vi "Create Oneof Message Converter Skeletons.vi"(8 "error in (no error)":errorcluster, 10 "Message parameters":T1[](array[typedef]), 11 "Library in":refnum<vi>) -> (0 "error out":errorcluster, 3 "Library out":refnum<vi>)   [LabVIEW 2025, in "gRPC Template Creation Utility.lvlib"]
uses:
  gRPC Template Creation Utility.lvlib
  TypeDefs/Message Metadata (Scripting).ctl
  TypeDefs/Message Element Metadata (Scripting).ctl
  TypeDefs/Message Element Type.ctl
  OneOf Constants/OneOfConstantsEnum.ctl
  <vilib>/Utility/traverseref.llb/TRef TravTarget.ctl
  <vilib>/Utility/traverseref.llb/VI Scripting - Traverse.lvlib
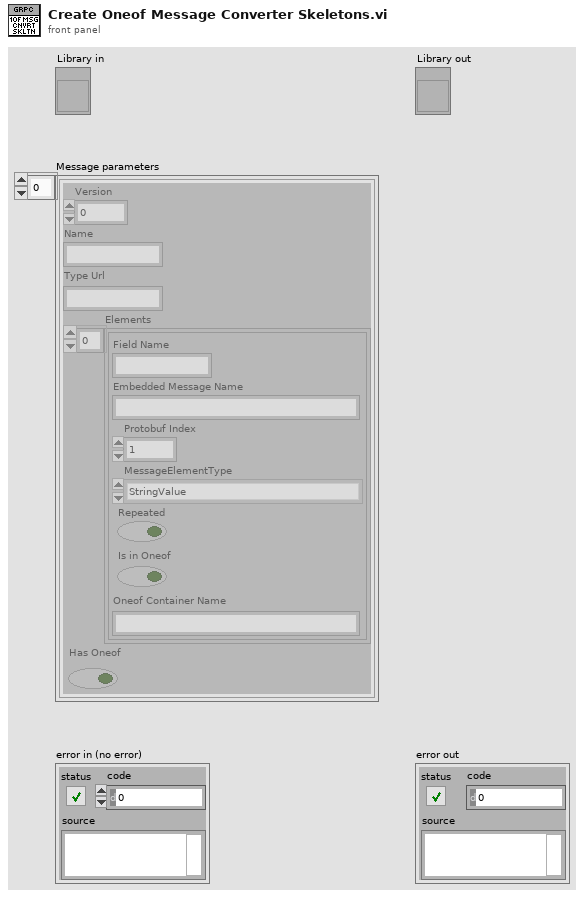
[diagram p1: front panel]
types:
  T1 = typedef "gRPC Template Creation Utility.lvlib/Message Metadata (Scripting).ctl" = cluster{"Version":i32, "Name":string, "Type Url":string, "Elements":T2[], "Has Oneof":bool}
  T2 = typedef "gRPC Template Creation Utility.lvlib/Message Element Metadata (Scripting).ctl" = cluster{"Field Name":string, "Embedded Message Name":string, "Protobuf Index":i32, "MessageElementType":T3, "Repeated":bool, "Is in Oneof":bool, "Oneof Container Name":string}
  T3 = typedef "gRPC Template Creation Utility.lvlib/Message Element Type.ctl" = enum32{"Int32Value", "FloatValue", "DoubleValue", "BoolValue", "StringValue", "MessageValue", "Int64Value", "UInt32Value", "UInt64Value", "EnumValue", "Bytes", "Fixed64", "Fixed32", "SFixed64", "SFixed32", "SInt64", "SInt32"}
  T4 = typedef "gRPC Template Creation Utility.lvlib/OneOfConstantsEnum.ctl" = enum16{"FlatToRichVIPrefix", "RichToFlatVIPrefix", "FlatTypeDefSuffix"}
  T5 = typedef "TRef TravTarget.ctl" = enum16{"FP", "BD", "Other"}
  T6 = enum32{"invalid scope", "public", "private", "protected", "community"}
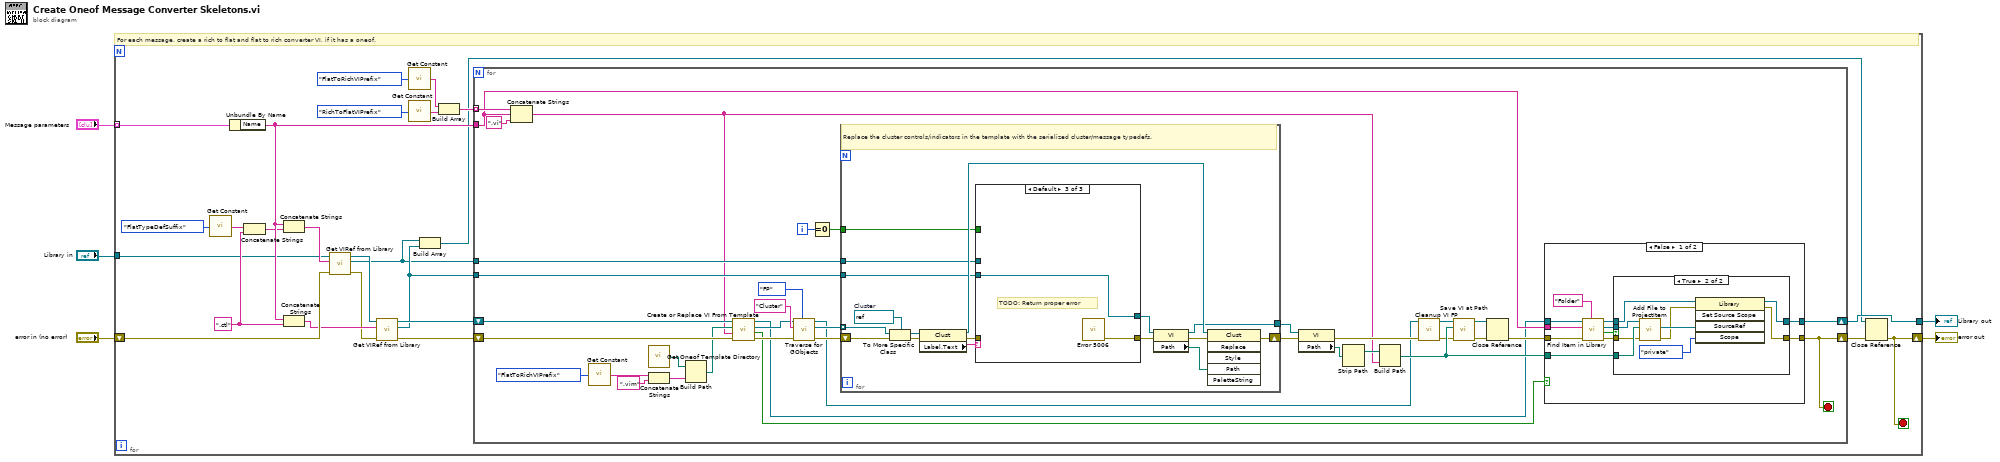
[diagram p0: block diagram]
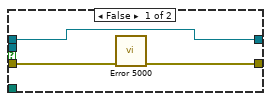
[diagram p2: hidden frame]
diagram:
  n1 = for {
    tunnel: "Message parameters" -> [w30] mode=indexing
    shift-right: [w7] -> w3
    shift-left: "error in (no error)" -> [w29]
    tunnel: "Library in" -> [w14]
    tunnel: [w27] -> w5
    stop <- w7 stop-if-true
    w15 = ".ctl" ("string")
    # "For each message, create a rich to flat and flat to rich converter VI, if it has a oneof."
    n2 = call "Get Constant.vi"("Selection"=OneOfConstantsEnum."FlatTypeDefSuffix") -> ("String"=w21:string)
    n3 = Unbundle By Name(w30) -> ("Name"=w24:string)
    n4 = Concatenate Strings(w21, w15) -> (w23:string)
    n5 = Concatenate Strings(w24, w23) -> (w26:string)
    n6 = Concatenate Strings(w24, w15) -> (w25:string)
    n7 = call "Get VIRef from Library.vi"("error in (no error)"=w29, "item name"=w26, "library in"=w14) -> ("error out"=w12:errorcluster, "vi"=w9:refnum<vi>, "library out"=w13:refnum<vi>)  [unwired: 5 in, 1 out]
    n8 = call "Get VIRef from Library.vi"("error in (no error)"=w12, "item name"=w25, "library in"=w13) -> ("error out"=w11:errorcluster, "vi"=w10:refnum<vi>, "library out"=w28:refnum<vi>)  [unwired: 5 in, 1 out]
    n9 = call "Get Constant.vi"("Selection"=OneOfConstantsEnum."FlatToRichVIPrefix") -> ("String"=w18:string)
    n10 = call "Get Constant.vi"("Selection"=OneOfConstantsEnum."RichToFlatVIPrefix") -> ("String"=w17:string)
    n11 = Build Array(w9, w10) -> (w6:refnum<vi>[])
    n12 = Build Array(w18, w17) -> (w16:string[])
    n13 = for {
      tunnel: w9 -> [w68]
      tunnel: w24 -> [w52]
      tunnel: w10 -> [w63]
      shift-right: [w40] -> w27
      shift-left: w28 -> [w35]
      shift-right: [w32] -> w8
      shift-left: w11 -> [w39]
      tunnel: w16 -> [w57] mode=indexing
      i -> [w56]
      stop <- w32 stop-if-true
      n14 = Concatenate Strings(w57, w52, ".vi" ("string")) -> (w33:string)
      n15 = call "Get Constant.vi"("Selection"=OneOfConstantsEnum."FlatToRichVIPrefix") -> ("String"=w50:string)
      n16 = call "Get Oneof Template Directory.vi"() -> ("appended path"=w53:path)
      n17 = Concatenate Strings(w50, ".vim" ("string")) -> (w48:string)
      n18 = Build Path(base path=w53, name or relative path=w48) -> (appended path=w34:path)
      n19 = call "Create or Replace VI From Template.vi"("error in (no error)"=w39, "vi name"=w33, "template vi path"=w34, "library in"=w35) -> ("error out"=w38:errorcluster, "existing vi"=w31:bool, "vi"=w37:refnum<vi>, "Library out"=w36:refnum<vi>)  [unwired: 4 in]
      n20 = call <vilib>:"Traverse for GObjects.vi"("Traverse Target"=TRef_TravTarget."FP", "error in (no error)"=w38, "Class Name"="Cluster", "VI Refnum"=w37) -> ("error out"=w58:errorcluster, "References"=w60:refnum<vi>[], "dup VI Refnum"=w45:refnum<vi>)  [unwired: 4 in, 1 out]
      n21 = Equal To 0?(x=w56) -> (x = 0?=w55:bool)
      n22 = for {
        tunnel: w60 -> [w101] mode=indexing
        tunnel: w68 -> [w105]
        tunnel: w63 -> [w104]
        shift-right: [w100] -> w59
        shift-left: w58 -> [w102]
        tunnel: [w99] -> w67
        tunnel: w55 -> [w94]
        w109 = refnum<vi> refnum  # Cluster
        # "Replace the cluster controls/indicators in the template with the serialized cluster/message typedefs."
        n23 = To More Specific Class(target class=w109, reference=w101, error in=w102) -> (specific class reference=w108:refnum<vi>, error out=w110:errorcluster)
        n24 = property class="Clust"(reference=w108, error in=w110) -> (reference out=w106:refnum<vi>, error out=w103:errorcluster, "Label.Text"=w107:string)
        n25 = case shown="Default" w107 {
          tunnel: w105 -> [w113 w121 _]
          tunnel: w104 -> [w112 w120 w125]
          tunnel: w103 -> [w115 w118 _]
          tunnel: [w111 w119 w125] -> w95
          tunnel: [w115 w118 w126] -> w96
          tunnel: w94 -> [w114 w122 _]
          frame "OutputCluster", "OutputClusterType" {
            n26 = case shown="True" w114 {
              tunnel: w113 -> [w116 _]
              tunnel: w112 -> [_ w117]
              tunnel: [w116 w117] -> w111
              frame False {
                # "Convert Class to Cluster. Wire flat cluster as output"
              }
              frame True {
                # "Convert Cluster to Class.\nWire rich cluster as output"
              }
            }
          }
          frame "InputCluster" {
            n27 = case shown="True" w122 {
              tunnel: w121 -> [_ w124]
              tunnel: w120 -> [w123 _]
              tunnel: [w123 w124] -> w119
              frame False {
                # "Convert Class to Cluster. Wire rich cluster as input."
              }
              frame True {
                # "Convert Cluster to Class. Wire flat cluster as input"
              }
            }
          }
          frame Default {
            # "TODO: Return proper error"
            n28 = call "Error 5006.vi"() -> ("error out"=w126:errorcluster)  [unwired: 11 in]
          }
        }
        n29 = property class="VI"(reference=w95, error in=w96) -> (reference out=w99:refnum<vi>, error out=w98:errorcluster, "Path"=w97:path)
        n30 = invoke class="Clust" method="Replace"(reference=w106, error in=w98, "Path"=w97) -> (error out=w100:errorcluster)  [unwired: 3 in, 5 out]
      }
      n31 = property class="VI"(reference=w67, error in=w59) -> (error out=w47:errorcluster, "Path"=w66:path)  [unwired: 1 out]
      n32 = Strip Path(path=w66) -> (stripped path=w65:path)  [unwired: 1 out]
      n33 = Build Path(base path=w65, name or relative path=w33) -> (appended path=w54:path)
      n34 = call "Cleanup VI FP.vi"("error in"=w47, "vi in"=w45) -> ("error out"=w46:errorcluster, "vi out"=w44:refnum<vi>)  [unwired: 8 in]
      n35 = call "Save VI at Path.vi"("error in (no error)"=w46, "Path"=w54, "VI in"=w44) -> ("error out"=w43:errorcluster, "VI out"=w42:refnum<vi>)  [unwired: 6 in, 1 out]
      n36 = Close Reference(reference=w42, error in (no error)=w43) -> (error out=w41:errorcluster)
      n37 = case shown="False" w31 {
        tunnel: w54 -> [w77 _]
        tunnel: w52 -> [w74 _]
        tunnel: w41 -> [w73 w93]
        tunnel: [w71 w92] -> w40
        tunnel: w36 -> [w70 w92]
        tunnel: [w69 w93] -> w32
        frame False {
          n38 = call "Find Item in Library.vi"("Item Type"="Folder", "error in (no error)"=w73, "Item Name"=w74, "Library item in"=w70) -> ("error out"=w76:errorcluster, "Found?"=w75:bool, "Project Item (Library Item)"=w78:refnum<vi>, "Library item out"=w72:refnum<vi>)  [unwired: 4 in]
          n39 = case shown="True" w75 {
            tunnel: w78 -> [_ w91]
            tunnel: w77 -> [_ w90]
            tunnel: w76 -> [w81 w89]
            tunnel: [w80 w84] -> w69
            tunnel: w72 -> [w82 w88]
            tunnel: [w82 w86] -> w71
            frame False {
              n40 = call "Error 5000.vi"("error in (no error)"=w81) -> ("error out"=w80:errorcluster)  [unwired: 10 in]
            }
            frame True {
              n41 = call "Add File to ProjectItem.vi"("error in (no error)"=w89, "File Path"=w90, "ProjectItem in"=w91) -> ("error out"=w85:errorcluster, "Added File ref"=w87:refnum<vi>)  [unwired: 6 in, 1 out]
              n42 = invoke class="Library" method="Set Source Scope"(reference=w88, error in=w85, "SourceRef"=w87, "Scope"=T6."private" ("scope")) -> (reference out=w86:refnum<vi>, error out=w84:errorcluster)  [unwired: 1 in, 3 out]
            }
          }
        }
        frame True {
        }
      }
    }
    n43 = Close Reference(reference=w6, error in (no error)=w8) -> (error out=w7:errorcluster)
  }
  "Library out" <- w5
  "error out" <- w3
